vi "Parameter Filter - By Core Number.vi"(2 "Core Number":i32, 7 "Parameters Array (in)":T1[](array[typedef])) -> (8 "Filtered Parameters Array (out)":T1[](array[typedef]))   [LabVIEW 2017] (continued)
 "Scale"="0.5", "Offset"="0", "Signed"=TRUE, "Unit"="Deg C", "Encoding"=enum."BNR", "Default Value"="0"}, {"Core Number"=0, "Channel Number"=7, "Channel Name"="RDC18_ENG_RB1", "Channel Speed"=100, "Label Decimal"=189, "Label Name"="Label_275", "Min Rate (mS)"=800, "Max Rate (mS)"=1200, "SDI"=3, "SSM"=3, "Create SDI"=FALSE, "Create SSM"=FALSE, "Create Parity"=FALSE, "Parameter Name"="rdc18_eng_rb1_lbl275_b18_28", "Start Bit"=18, "Number of Bits"=11, "Scale"="0.5", "Offset"="0", "Signed"=TRUE, "Unit"="Deg C", "Encoding"=enum."BNR", "Default Value"="0"}, {"Core Number"=0, "Channel Number"=7, "Channel Name"="RDC18_ENG_RB1", "Channel Speed"=100, "Label Decimal"=184, "Label Name"="Label_270", "Min Rate (mS)"=80, "Max Rate (mS)"=120, "SDI"=3, "SSM"=0, "Create SDI"=FALSE, "Create SSM"=FALSE, "Create Parity"=FALSE, "Parameter Name"="rdc18_eng_rb1_lbl270_b10_28", "Start Bit"=10, "Number of Bits"=19, "Scale"="1", "Offset"="0", "Signed"=FALSE, "Unit"="N/A", "Encoding"=enum."Discrete", "Default Value"="0"}, {"Core Number"=0, "Channel Number"=7, "Channel Name"="RDC18_ENG_RB1", "Channel Speed"=100, "Label Decimal"=185, "Label Name"="Label_271", "Min Rate (mS)"=80, "Max Rate (mS)"=120, "SDI"=3, "SSM"=0, "Create SDI"=FALSE, "Create SSM"=FALSE, "Create Parity"=FALSE, "Parameter Name"="rdc18_eng_rb1_lbl271_b10_28", "Start Bit"=10, "Number of Bits"=19, "Scale"="1", "Offset"="0", "Signed"=FALSE, "Unit"="N/A", "Encoding"=enum."Discrete", "Default Value"="0"}, {"Core Number"=0, "Channel Number"=7, "Channel Name"="RDC18_ENG_RB1", "Channel Speed"=100, "Label Decimal"=186, "Label Name"="Label_272", "Min Rate (mS)"=80, "Max Rate (mS)"=120, "SDI"=3, "SSM"=0, "Create SDI"=FALSE, "Create SSM"=FALSE, "Create Parity"=FALSE, "Parameter Name"="rdc18_eng_rb1_lbl272_b10_28", "Start Bit"=10, "Number of Bits"=19, "Scale"="1", "Offset"="0", "Signed"=FALSE, "Unit"="N/A", "Encoding"=enum."Discrete", "Default Value"="0"}, {"Core Number"=0, "Channel Number"=7, "Channel Name"="RDC18_ENG_RB1", "Channel Speed"=100, "Label Decimal"=187, "Label Name"="Label_273", "Min Rate (mS)"=80, "Max Rate (mS)"=120, "SDI"=3, "SSM"=0, "Create SDI"=FALSE, "Create SSM"=FALSE, "Create Parity"=FALSE, "Parameter Name"="rdc18_eng_rb1_lbl273_b10_28", "Start Bit"=10, "Number of Bits"=19, "Scale"="1", "Offset"="0", "Signed"=FALSE, "Unit"="N/A", "Encoding"=enum."Discrete", "Default Value"="0"}, {"Core Number"=0, "Channel Number"=7, "Channel Name"="RDC18_ENG_RB1", "Channel Speed"=100, "Label Decimal"=151, "Label Name"="Label_227", "Min Rate (mS)"=80, "Max Rate (mS)"=120, "SDI"=3, "SSM"=0, "Create SDI"=FALSE, "Create SSM"=FALSE, "Create Parity"=FALSE, "Parameter Name"="rdc18_eng_rb1_lbl227_b10_28", "Start Bit"=10, "Number of Bits"=19, "Scale"="1", "Offset"="0", "Signed"=FALSE, "Unit"="N/A", "Encoding"=enum."Discrete", "Default Value"="0"}, {"Core Number"=0, "Channel Number"=7, "Channel Name"="RDC18_ENG_RB1", "Channel Speed"=100, "Label Decimal"=105, "Label Name"="Label_151", "Min Rate (mS)"=800, "Max Rate (mS)"=1200, "SDI"=3, "SSM"=0, "Create SDI"=FALSE, "Create SSM"=FALSE, "Create Parity"=FALSE, "Parameter Name"="rdc18_eng_rb1_lbl151_b10_27", "Start Bit"=10, "Number of Bits"=18, "Scale"="1", "Offset"="0", "Signed"=FALSE, "Unit"="N/A", "Encoding"=enum."Discrete", "Default Value"="0"}, {"Core Number"=0, "Channel Number"=8, "Channel Name"="RDC18_ENG_RB2", "Channel Speed"=100, "Label Decimal"=213, "Label Name"="Label_325", "Min Rate (mS)"=40, "Max Rate (mS)"=60, "SDI"=3, "SSM"=3, "Create SDI"=FALSE, "Create SSM"=FALSE, "Create Parity"=FALSE, "Parameter Name"="rdc18_eng_rb2_lbl325_b10_28", "Start Bit"=10, "Number of Bits"=19, "Scale"="0.0006866", "Offset"="0", "Signed"=TRUE, "Unit"="Degrees", "Encoding"=enum."BNR", "Default Value"="0"}, {"Core Number"=0, "Channel Number"=8, "Channel Name"="RDC18_ENG_RB2", "Channel Speed"=100, "Label Decimal"=91, "Label Name"="Label_133", "Min Rate (mS)"=40, "Max Rate (mS)"=60, "SDI"=3, "SSM"=3, "Create SDI"=FALSE, "Create SSM"=FALSE, "Create Parity"=FALSE, "Parameter Name"="rdc18_eng_rb2_lbl133_b10_28", "Start Bit"=10, "Number of Bits"=19, "Scale"="0.0006866", "Offset"="0", "Signed"=TRUE, "Unit"="Degrees", "Encoding"=enum."BNR", "Default Value"="0"}, {"Core Number"=0, "Channel Number"=8, "Channel Name"="RDC18_ENG_RB2", "Channel Speed"=100, "Label Decimal"=104, "Label Name"="Label_150", "Min Rate (mS)"=800, "Max Rate (mS)"=1200, "SDI"=3, "SSM"=3, "Create SDI"=FALSE, "Create SSM"=FALSE, "Create Parity"=FALSE, "Parameter Name"="rdc18_eng_rb2_lbl150_b11_27", "Start Bit"=11, "Number of Bits"=17, "Scale"="1", "Offset"="0", "Signed"=FALSE, "Unit"="hh.mm.ss", "Encoding"=enum."BNR", "Default Value"="0"}, {"Core Number"=0, "Channel Number"=8, "Channel Name"="RDC18_ENG_RB2", "Channel Speed"=100, "Label Decimal"=39, "Label Name"="Label_47", "Min Rate (mS)"=800, "Max Rate (mS)"=1200, "SDI"=3, "SSM"=3, "Create SDI"=FALSE, "Create SSM"=FALSE, "Create Parity"=FALSE, "Parameter Name"="rdc18_eng_rb2_lbl47_b10_27", "Start Bit"=10, "Number of Bits"=18, "Scale"="1", "Offset"="0", "Signed"=FALSE, "Unit"="N/A", "Encoding"=enum."BNR", "Default Value"="0"}, {"Core Number"=0, "Channel Number"=8, "Channel Name"="RDC18_ENG_RB2", "Channel Speed"=100, "Label Decimal"=188, "Label Name"="Label_274", "Min Rate (mS)"=800, "Max Rate (mS)"=1200, "SDI"=3, "SSM"=3, "Create SDI"=FALSE, "Create SSM"=FALSE, "Create Parity"=FALSE, "Parameter Name"="rdc18_eng_rb2_lbl274_b18_28", "Start Bit"=18, "Number of Bits"=11, "Scale"="0.5", "Offset"="0", "Signed"=TRUE, "Unit"="Deg C", "Encoding"=enum."BNR", "Default Value"="0"}, {"Core Number"=0, "Channel Number"=8, "Channel Name"="RDC18_ENG_RB2", "Channel Speed"=100, "Label Decimal"=189, "Label Name"="Label_275", "Min Rate (mS)"=800, "Max Rate (mS)"=1200, "SDI"=3, "SSM"=3, "Create SDI"=FALSE, "Create SSM"=FALSE, "Create Parity"=FALSE, "Parameter Name"="rdc18_eng_rb2_lbl275_b18_28", "Start Bit"=18, "Number of Bits"=11, "Scale"="0.5", "Offset"="0", "Signed"=TRUE, "Unit"="Deg C", "Encoding"=enum."BNR", "Default Value"="0"}, {"Core Number"=0, "Channel Number"=8, "Channel Name"="RDC18_ENG_RB2", "Channel Speed"=100, "Label Decimal"=184, "Label Name"="Label_270", "Min Rate (mS)"=80, "Max Rate (mS)"=120, "SDI"=3, "SSM"=0, "Create SDI"=FALSE, "Create SSM"=FALSE, "Create Parity"=FALSE, "Parameter Name"="rdc18_eng_rb2_lbl270_b10_28", "Start Bit"=10, "Number of Bits"=19, "Scale"="1", "Offset"="0", "Signed"=FALSE, "Unit"="N/A", "Encoding"=enum."Discrete", "Default Value"="0"}, {"Core Number"=0, "Channel Number"=8, "Channel Name"="RDC18_ENG_RB2", "Channel Speed"=100, "Label Decimal"=185, "Label Name"="Label_271", "Min Rate (mS)"=80, "Max Rate (mS)"=120, "SDI"=3, "SSM"=0, "Create SDI"=FALSE, "Create SSM"=FALSE, "Create Parity"=FALSE, "Parameter Name"="rdc18_eng_rb2_lbl271_b10_28", "Start Bit"=10, "Number of Bits"=19, "Scale"="1", "Offset"="0", "Signed"=FALSE, "Unit"="N/A", "Encoding"=enum."Discrete", "Default Value"="0"}, {"Core Number"=0, "Channel Number"=8, "Channel Name"="RDC18_ENG_RB2", "Channel Speed"=100, "Label Decimal"=186, "Label Name"="Label_272", "Min Rate (mS)"=80, "Max Rate (mS)"=120, "SDI"=3, "SSM"=0, "Create SDI"=FALSE, "Create SSM"=FALSE, "Create Parity"=FALSE, "Parameter Name"="rdc18_eng_rb2_lbl272_b10_28", "Start Bit"=10, "Number of Bits"=19, "Scale"="1", "Offset"="0", "Signed"=FALSE, "Unit"="N/A", "Encoding"=enum."Discrete", "Default Value"="0"}, {"Core Number"=0, "Channel Number"=8, "Channel Name"="RDC18_ENG_RB2", "Channel Speed"=100, "Label Decimal"=187, "Label Name"="Label_273", "Min Rate (mS)"=80, "Max Rate (mS)"=120, "SDI"=3, "SSM"=0, "Create SDI"=FALSE, "Create SSM"=FALSE, "Create Parity"=FALSE, "Parameter Name"="rdc18_eng_rb2_lbl273_b10_28", "Start Bit"=10, "Number of Bits"=19, "Scale"="1", "Offset"="0", "Signed"=FALSE, "Unit"="N/A", "Encoding"=enum."Discrete", "Default Value"="0"}, {"Core Number"=0, "Channel Number"=8, "Channel Name"="RDC18_ENG_RB2", "Channel Speed"=100, "Label Decimal"=151, "Label Name"="Label_227", "Min Rate (mS)"=80, "Max Rate (mS)"=120, "SDI"=3, "SSM"=0, "Create SDI"=FALSE, "Create SSM"=FALSE, "Create Parity"=FALSE, "Parameter Name"="rdc18_eng_rb2_lbl227_b10_28", "Start Bit"=10, "Number of Bits"=19, "Scale"="1", "Offset"="0", "Signed"=FALSE, "Unit"="N/A", "Encoding"=enum."Discrete", "Default Value"="0"}, {"Core Number"=0, "Channel Number"=8, "Channel Name"="RDC18_ENG_RB2", "Channel Speed"=100, "Label Decimal"=105, "Label Name"="Label_151", "Min Rate (mS)"=800, "Max Rate (mS)"=1200, "SDI"=3, "SSM"=0, "Create SDI"=FALSE, "Create SSM"=FALSE, "Create Parity"=FALSE, "Parameter Name"="rdc18_eng_rb2_lbl151_b10_27", "Start Bit"=10, "Number of Bits"=18, "Scale"="1", "Offset"="0", "Signed"=FALSE, "Unit"="N/A", "Encoding"=enum."Discrete", "Default Value"="0"}, {"Core Number"=0, "Channel Number"=27, "Channel Name"="LGCS_MON2_TX", "Channel Speed"=100, "Label Decimal"=17, "Label Name"="Label_21", "Min Rate (mS)"=10, "Max Rate (mS)"=30, "SDI"=0, "SSM"=0, "Create SDI"=FALSE, "Create SSM"=FALSE, "Create Parity"=FALSE, "Parameter Name"="m2_dnlk_status_msg", "Start Bit"=8, "Number of Bits"=23, "Scale"="1", "Offset"="0", "Signed"=FALSE, "Unit"="", "Encoding"=enum."BNR", "Default Value"="0"}, {"Core Number"=0, "Channel Number"=27, "Channel Name"="LGCS_MON2_TX", "Channel Speed"=100, "Label Decimal"=18, "Label Name"="Label_22", "Min Rate (mS)"=10, "Max Rate (mS)"=30, "SDI"=0, "SSM"=0, "Create SDI"=FALSE, "Create SSM"=FALSE, "Create Parity"=FALSE, "Parameter Name"="m2_consilidated_wow_status", "Start Bit"=8, "Number of Bits"=23, "Scale"="1", "Offset"="0", "Signed"=FALSE, "Unit"="", "Encoding"=enum."BNR", "Default Value"="0"}, {"Core Number"=0, "Channel Number"=27, "Channel Name"="LGCS_MON2_TX", "Channel Speed"=100, "Label Decimal"=19, "Label Name"="Label_23", "Min Rate (mS)"=80, "Max Rate (mS)"=120, "SDI"=3, "SSM"=0, "Create SDI"=FALSE, "Create SSM"=FALSE, "Create Parity"=FALSE, "Parameter Name"="baulk_solenoid_ctl_ch1", "Start Bit"=26, "Number of Bits"=1, "Scale"="0", "Offset"="0", "Signed"=FALSE, "Unit"="", "Encoding"=enum."Discrete", "Default Value"="0"}, {"Core Number"=0, "Channel Number"=27, "Channel Name"="LGCS_MON2_TX", "Channel Speed"=100, "Label Decimal"=19, "Label Name"="Label_23", "Min Rate (mS)"=80, "Max Rate (mS)"=120, "SDI"=3, "SSM"=0, "Create SDI"=FALSE, "Create SSM"=FALSE, "Create Parity"=FALSE, "Parameter Name"="baulk_solenoid_ctl_ch2", "Start Bit"=27, "Number of Bits"=1, "Scale"="0", "Offset"="0", "Signed"=FALSE, "Unit"="", "Encoding"=enum."Discrete", "Default Value"="0"}, {"Core Number"=0, "Channel Number"=27, "Channel Name"="LGCS_MON2_TX", "Channel Speed"=100, "Label Decimal"=19, "Label Name"="Label_23", "Min Rate (mS)"=80, "Max Rate (mS)"=120, "SDI"=3, "SSM"=0, "Create SDI"=FALSE, "Create SSM"=FALSE, "Create Parity"=FALSE, "Parameter Name"="mlg_doors_close_highside_solenoid_driver_ctl_ch1", "Start Bit"=17, "Number of Bits"=1, "Scale"="0", "Offset"="0", "Signed"=FALSE, "Unit"="", "Encoding"=enum."Discrete", "Default Value"="0"}, {"Core Number"=0, "Channel Number"=27, "Channel Name"="LGCS_MON2_TX", "Channel Speed"=100, "Label Decimal"=19, "Label Name"="Label_23", "Min Rate (mS)"=80, "Max Rate (mS)"=120, "SDI"=3, "SSM"=0, "Create SDI"=FALSE, "Create SSM"=FALSE, "Create Parity"=FALSE, "Parameter Name"="mlg_doors_close_highside_solenoid_driver_ctl_ch2", "Start Bit"=25, "Number of Bits"=1, "Scale"="0", "Offset"="0", "Signed"=FALSE, "Unit"="", "Encoding"=enum."Discrete", "Default Value"="0"}, {"Core Number"=0, "Channel Number"=27, "Channel Name"="LGCS_MON2_TX", "Channel Speed"=100, "Label Decimal"=19, "Label Name"="Label_23", "Min Rate (mS)"=80, "Max Rate (mS)"=120, "SDI"=3, "SSM"=0, "Create SDI"=FALSE, "Create SSM"=FALSE, "Create Parity"=FALSE, "Parameter Name"="mlg_doors_close_lowside_solenoid_driver_ctl_ch1", "Start Bit"=16, "Number of Bits"=1, "Scale"="0", "Offset"="0", "Signed"=FALSE, "Unit"="", "Encoding"=enum."Discrete", "Default Value"="0"}, {"Core Number"=0, "Channel Number"=27, "Channel Name"="LGCS_MON2_TX", "Channel Speed"=100, "Label Decimal"=19, "Label Name"="Label_23", "Min Rate (mS)"=80, "Max Rate (mS)"=120, "SDI"=3, "SSM"=0, "Create SDI"=FALSE, "Create SSM"=FALSE, "Create Parity"=FALSE, "Parameter Name"="mlg_doors_close_lowside_solenoid_driver_ctl_ch2", "Start Bit"=24, "Number of Bits"=1, "Scale"="0", "Offset"="0", "Signed"=FALSE, "Unit"="", "Encoding"=enum."Discrete", "Default Value"="0"}, {"Core Number"=0, "Channel Number"=27, "Channel Name"="LGCS_MON2_TX", "Channel Speed"=100, "Label Decimal"=19, "Label Name"="Label_23", "Min Rate (mS)"=80, "Max Rate (mS)"=120, "SDI"=3, "SSM"=0, "Create SDI"=FALSE, "Create SSM"=FALSE, "Create Parity"=FALSE, "Parameter Name"="mlg_doors_open_highside_solenoid_driver_ctl_ch1", "Start Bit"=15, "Number of Bits"=1, "Scale"="0", "Offset"="0", "Signed"=FALSE, "Unit"="", "Encoding"=enum."Discrete", "Default Value"="0"}, {"Core Number"=0, "Channel Number"=27, "Channel Name"="LGCS_MON2_TX", "Channel Speed"=100, "Label Decimal"=19, "Label Name"="Label_23", "Min Rate (mS)"=80, "Max Rate (mS)"=120, "SDI"=3, "SSM"=0, "Create SDI"=FALSE, "Create SSM"=FALSE, "Create Parity"=FALSE, "Parameter Name"="mlg_doors_open_highside_solenoid_driver_ctl_ch2", "Start Bit"=23, "Number of Bits"=1, "Scale"="0", "Offset"="0", "Signed"=FALSE, "Unit"="", "Encoding"=enum."Discrete", "Default Value"="0"}, {"Core Number"=0, "Channel Number"=27, "Channel Name"="LGCS_MON2_TX", "Channel Speed"=100, "Label Decimal"=19, "Label Name"="Label_23", "Min Rate (mS)"=80, "Max Rate (mS)"=120, "SDI"=3, "SSM"=0, "Create SDI"=FALSE, "Create SSM"=FALSE, "Create Parity"=FALSE, "Parameter Name"="mlg_doors_open_lowside_solenoid_driver_ctl_ch1", "Start Bit"=14, "Number of Bits"=1, "Scale"="0", "Offset"="0", "Signed"=FALSE, "Unit"="", "Encoding"=enum."Discrete", "Default Value"="0"}, {"Core Number"=0, "Channel Number"=27, "Channel Name"="LGCS_MON2_TX", "Channel Speed"=100, "Label Decimal"=19, "Label Name"="Label_23", "Min Rate (mS)"=80, "Max Rate (mS)"=120, "SDI"=3, "SSM"=0, "Create SDI"=FALSE, "Create SSM"=FALSE, "Create Parity"=FALSE, "Parameter Name"="mlg_doors_open_lowside_solenoid_driver_ctl_ch2", "Start Bit"=22, "Number of Bits"=1, "Scale"="0", "Offset"="0", "Signed"=FALSE, "Unit"="", "Encoding"=enum."Discrete", "Default Value"="0"}, {"Core Number"=0, "Channel Number"=27, "Channel Name"="LGCS_MON2_TX", "Channel Speed"=100, "Label Decimal"=19, "Label Name"="Label_23", "Min Rate (mS)"=80, "Max Rate (mS)"=120, "SDI"=3, "SSM"=0, "Create SDI"=FALSE, "Create SSM"=FALSE, "Create Parity"=FALSE, "Parameter Name"="mlg_extend_highsidesolenoiddriver_ctl_ch1", "Start Bit"=13, "Number of Bits"=1, "Scale"="0", "Offset"="0", "Signed"=FALSE, "Unit"="", "Encoding"=enum."Discrete", "Default Value"="0"}, {"Core Number"=0, "Channel Number"=27, "Channel Name"="LGCS_MON2_TX", "Channel Speed"=100, "Label Decimal"=19, "Label Name"="Label_23", "Min Rate (mS)"=80, "Max Rate (mS)"=120, "SDI"=3, "SSM"=0, "Create SDI"=FALSE, "Create SSM"=FALSE, "Create Parity"=FALSE, "Parameter Name"="mlg_extend_highsidesolenoiddriver_ctl_ch2", "Start Bit"=21, "Number of Bits"=1, "Scale"="0", "Offset"="0", "Signed"=FALSE, "Unit"="", "Encoding"=enum."Discrete", "Default Value"="0"}, {"Core Number"=0, "Channel Number"=27, "Channel Name"="LGCS_MON2_TX", "Channel Speed"=100, "Label Decimal"=19, "Label Name"="Label_23", "Min Rate (mS)"=80, "Max Rate (mS)"=120, "SDI"=3, "SSM"=0, "Create SDI"=FALSE, "Create SSM"=FALSE, "Create Parity"=FALSE, "Parameter Name"="mlg_extend_lowsidesolenoiddriver_ctl_ch1", "Start Bit"=12, "Number of Bits"=1, "Scale"="0", "Offset"="0", "Signed"=FALSE, "Unit"="", "Encoding"=enum."Discrete", "Default Value"="0"}, {"Core Number"=0, "Channel Number"=27, "Channel Name"="LGCS_MON2_TX", "Channel Speed"=100, "Label Decimal"=19, "Label Name"="Label_23", "Min Rate (mS)"=80, "Max Rate (mS)"=120, "SDI"=3, "SSM"=0, "Create SDI"=FALSE, "Create SSM"=FALSE, "Create Parity"=FALSE, "Parameter Name"="mlg_extend_lowsidesolenoiddriver_ctl_ch2", "Start Bit"=20, "Number of Bits"=1, "Scale"="0", "Offset"="0", "Signed"=FALSE, "Unit"="", "Encoding"=enum."Discrete", "Default Value"="0"}, {"Core Number"=0, "Channel Number"=27, "Channel Name"="LGCS_MON2_TX", "Channel Speed"=100, "Label Decimal"=19, "Label Name"="Label_23", "Min Rate (mS)"=80, "Max Rate (mS)"=120, "SDI"=3, "SSM"=0, "Create SDI"=FALSE, "Create SSM"=FALSE, "Create Parity"=FALSE, "Parameter Name"="mlg_retract_highsidesolenoiddriver_ctl_ch1", "Start Bit"=11, "Number of Bits"=1, "Scale"="0", "Offset"="0", "Signed"=FALSE, "Unit"="", "Encoding"=enum."Discrete", "Default Value"="0"}, {"Core Number"=0, "Channel Number"=27, "Channel Name"="LGCS_MON2_TX", "Channel Speed"=100, "Label Decimal"=19, "Label Name"="Label_23", "Min Rate (mS)"=80, "Max Rate (mS)"=120, "SDI"=3, "SSM"=0, "Create SDI"=FALSE, "Create SSM"=FALSE, "Create Parity"=FALSE, "Parameter Name"="mlg_retract_highsidesolenoiddriver_ctl_ch2", "Start Bit"=19, "Number of Bits"=1, "Scale"="0", "Offset"="0", "Signed"=FALSE, "Unit"="", "Encoding"=enum."Discrete", "Default Value"="0"}, {"Core Number"=0, "Channel Number"=27, "Channel Name"="LGCS_MON2_TX", "Channel Speed"=100, "Label Decimal"=19, "Label Name"="Label_23", "Min Rate (mS)"=80, "Max Rate (mS)"=120, "SDI"=3, "SSM"=0, "Create SDI"=FALSE, "Create SSM"=FALSE, "Create Parity"=FALSE, "Parameter Name"="mlg_retract_lowsidesolenoiddriver_ctl_ch1", "Start Bit"=10, "Number of Bits"=1, "Scale"="0", "Offset"="0", "Signed"=FALSE, "Unit"="", "Encoding"=enum."Discrete", "Default Value"="0"}, {"Core Number"=0, "Channel Number"=27, "Channel Name"="LGCS_MON2_TX", "Channel Speed"=100, "Label Decimal"=19, "Label Name"="Label_23", "Min Rate (mS)"=80, "Max Rate (mS)"=120, "SDI"=3, "SSM"=0, "Create SDI"=FALSE, "Create SSM"=FALSE, "Create Parity"=FALSE, "Parameter Name"="mlg_retract_lowsidesolenoiddriver_ctl_ch2", "Start Bit"=18, "Number of Bits"=1, "Scale"="0", "Offset"="0", "Signed"=FALSE, "Unit"="", "Encoding"=enum."Discrete", "Default Value"="0"}, {"Core Number"=0, "Channel Number"=27, "Channel Name"="LGCS_MON2_TX", "Channel Speed"=100, "Label Decimal"=20, "Label Name"="Label_24", "Min Rate (mS)"=80, "Max Rate (mS)"=120, "SDI"=0, "SSM"=0, "Create SDI"=FALSE, "Create SSM"=FALSE, "Create Parity"=FALSE, "Parameter Name"="m1_m2_cas_msg", "Start Bit"=8, "Number of Bits"=23, "Scale"="1", "Offset"="0", "Signed"=FALSE, "Unit"="", "Encoding"=enum."BNR", "Default Value"="0"}, {"Core Number"=0, "Channel Number"=27, "Channel Name"="LGCS_MON2_TX", "Channel Speed"=100, "Label Decimal"=21, "Label Name"="Label_25", "Min Rate (mS)"=80, "Max Rate (mS)"=120, "SDI"=3, "SSM"=0, "Create SDI"=FALSE, "Create SSM"=FALSE, "Create Parity"=FALSE, "Parameter Name"="baulk_solenoid_ctl_ch1", "Start Bit"=26, "Number of Bits"=1, "Scale"="0", "Offset"="0", "Signed"=FALSE, "Unit"="", "Encoding"=enum."Discrete", "Default Value"="0"}, {"Core Number"=0, "Channel Number"=27, "Channel Name"="LGCS_MON2_TX", "Channel Speed"=100, "Label Decimal"=21, "Label Name"="Label_25", "Min Rate (mS)"=80, "Max Rate (mS)"=120, "SDI"=3, "SSM"=0, "Create SDI"=FALSE, "Create SSM"=FALSE, "Create Parity"=FALSE, "Parameter Name"="baulk_solenoid_ctl_ch2", "Start Bit"=27, "Number of Bits"=1, "Scale"="0", "Offset"="0", "Signed"=FALSE, "Unit"="", "Encoding"=enum."Discrete", "Default Value"="0"}, {"Core Number"=0, "Channel Number"=27, "Channel Name"="LGCS_MON2_TX", "Channel Speed"=100, "Label Decimal"=21, "Label Name"="Label_25", "Min Rate (mS)"=80, "Max Rate (mS)"=120, "SDI"=3, "SSM"=0, "Create SDI"=FALSE, "Create SSM"=FALSE, "Create Parity"=FALSE, "Parameter Name"="nlg_doors_close_highside_solenoid_driver_ctl_ch1", "Start Bit"=17, "Number of Bits"=1, "Scale"="0", "Offset"="0", "Signed"=FALSE, "Unit"="", "Encoding"=enum."Discrete", "Default Value"="0"}, {"Core Number"=0, "Channel Number"=27, "Channel Name"="LGCS_MON2_TX", "Channel Speed"=100, "Label Decimal"=21, "Label Name"="Label_25", "Min Rate (mS)"=80, "Max Rate (mS)"=120, "SDI"=3, "SSM"=0, "Create SDI"=FALSE, "Create SSM"=FALSE, "Create Parity"=FALSE, "Parameter Name"="nlg_doors_close_highside_solenoid_driver_ctl_ch2", "Start Bit"=25, "Number of Bits"=1, "Scale"="0", "Offset"="0", "Signed"=FALSE, "Unit"="", "Encoding"=enum."Discrete", "Default Value"="0"}, {"Core Number"=0, "Channel Number"=27, "Channel Name"="LGCS_MON2_TX", "Channel Speed"=100, "Label Decimal"=21, "Label Name"="Label_25", "Min Rate (mS)"=80, "Max Rate (mS)"=120, "SDI"=3, "SSM"=0, "Create SDI"=FALSE, "Create SSM"=FALSE, "Create Parity"=FALSE, "Parameter Name"="nlg_doors_close_lowside_solenoid_driver_ctl_ch1", "Start Bit"=16, "Number of Bits"=1, "Scale"="0", "Offset"="0", "Signed"=FALSE, "Unit"="", "Encoding"=enum."Discrete", "Default Value"="0"}, {"Core Number"=0, "Channel Number"=27, "Channel Name"="LGCS_MON2_TX", "Channel Speed"=100, "Label Decimal"=21, "Label Name"="Label_25", "Min Rate (mS)"=80, "Max Rate (mS)"=120, "SDI"=3, "SSM"=0, "Create SDI"=FALSE, "Create SSM"=FALSE, "Create Parity"=FALSE, "Parameter Name"="nlg_doors_close_lowside_solenoid_driver_ctl_ch2", "Start Bit"=24, "Number of Bits"=1, "Scale"="0", "Offset"="0", "Signed"=FALSE, "Unit"="", "Encoding"=enum."Discrete", "Default Value"="0"}, {"Core Number"=0, "Channel Number"=27, "Channel Name"="LGCS_MON2_TX", "Channel Speed"=100, "Label Decimal"=21, "Label Name"="Label_25", "Min Rate (mS)"=80, "Max Rate (mS)"=120, "SDI"=3, "SSM"=0, "Create SDI"=FALSE, "Create SSM"=FALSE, "Create Parity"=FALSE, "Parameter Name"="nlg_doors_open_highside_solenoid_driver_ctl_ch1", "Start Bit"=15, "Number of Bits"=1, "Scale"="0", "Offset"="0", "Signed"=FALSE, "Unit"="", "Encoding"=enum."Discrete", "Default Value"="0"}, {"Core Number"=0, "Channel Number"=27, "Channel Name"="LGCS_MON2_TX", "Channel Speed"=100, "Label Decimal"=21, "Label Name"="Label_25", "Min Rate (mS)"=80, "Max Rate (mS)"=120, "SDI"=3, "SSM"=0, "Create SDI"=FALSE, "Create SSM"=FALSE, "Create Parity"=FALSE, "Parameter Name"="nlg_doors_open_highside_solenoid_driver_ctl_ch2", "Start Bit"=23, "Number of Bits"=1, "Scale"="0", "Offset"="0", "Signed"=FALSE, "Unit"="", "Encoding"=enum."Discrete", "Default Value"="0"}, {"Core Number"=0, "Channel Number"=27, "Channel Name"="LGCS_MON2_TX", "Channel Speed"=100, "Label Decimal"=21, "Label Name"="Label_25", "Min Rate (mS)"=80, "Max Rate (mS)"=120, "SDI"=3, "SSM"=0, "Create SDI"=FALSE, "Create SSM"=FALSE, "Create Parity"=FALSE, "Parameter Name"="nlg_doors_open_lowside_solenoid_driver_ctl_ch1", "Start Bit"=14, "Number of Bits"=1, "Scale"="0", "Offset"="0", "Signed"=FALSE, "Unit"="", "Encoding"=enum."Discrete", "Default Value"="0"}, {"Core Number"=0, "Channel Number"=27, "Channel Name"="LGCS_MON2_TX", "Channel Speed"=100, "Label Decimal"=21, "Label Name"="Label_25", "Min Rate (mS)"=80, "Max Rate (mS)"=120, "SDI"=3, "SSM"=0, "Create SDI"=FALSE, "Create SSM"=FALSE, "Create Parity"=FALSE, "Parameter Name"="nlg_doors_open_lowside_solenoid_driver_ctl_ch2", "Start Bit"=22, "Number of Bits"=1, "Scale"="0", "Offset"="0", "Signed"=FALSE, "Unit"="", "Encoding"=enum."Discrete", "Default Value"="0"}, {"Core Number"=0, "Channel Number"=27, "Channel Name"="LGCS_MON2_TX", "Channel Speed"=100, "Label Decimal"=21, "Label Name"="Label_25", "Min Rate (mS)"=80, "Max Rate (mS)"=120, "SDI"=3, "SSM"=0, "Create SDI"=FALSE, "Create SSM"=FALSE, "Create Parity"=FALSE, "Parameter Name"="nlg_extend_highsidesolenoiddriver_ctl_ch1", "Start Bit"=13, "Number of Bits"=1, "Scale"="0", "Offset"="0", "Signed"=FALSE, "Unit"="", "Encoding"=enum."Discrete", "Default Value"="0"}, {"Core Number"=0, "Channel Number"=27, "Channel Name"="LGCS_MON2_TX", "Channel Speed"=100, "Label Decimal"=21, "Label Name"="Label_25", "Min Rate (mS)"=80, "Max Rate (mS)"=120, "SDI"=3, "SSM"=0, "Create SDI"=FALSE, "Create SSM"=FALSE, "Create Parity"=FALSE, "Parameter Name"="nlg_extend_highsidesolenoiddriver_ctl_ch2", "Start Bit"=21, "Number of Bits"=1, "Scale"="0", "Offset"="0", "Signed"=FALSE, "Unit"="", "Encoding"=enum."Discrete", "Default Value"="0"}, {"Core Number"=0, "Channel Number"=27, "Channel Name"="LGCS_MON2_TX", "Channel Speed"=100, "Label Decimal"=21, "Label Name"="Label_25", "Min Rate (mS)"=80, "Max Rate (mS)"=120, "SDI"=3, "SSM"=0, "Create SDI"=FALSE, "Create SSM"=FALSE, "Create Parity"=FALSE, "Parameter Name"="nlg_extend_lowsidesolenoiddriver_ctl_ch1", "Start Bit"=12, "Number of Bits"=1, "Scale"="0", "Offset"="0", "Signed"=FALSE, "Unit"="", "Encoding"=enum."Discrete", "Default Value"="0"}, {"Core Number"=0, "Channel Number"=27, "Channel Name"="LGCS_MON2_TX", "Channel Speed"=100, "Label Decimal"=21, "Label Name"="Label_25", "Min Rate (mS)"=80, "Max Rate (mS)"=120, "SDI"=3, "SSM"=0, "Create SDI"=FALSE, "Create SSM"=FALSE, "Create Parity"=FALSE, "Parameter Name"="nlg_extend_lowsidesolenoiddriver_ctl_ch2", "Start Bit"=20, "Number of Bits"=1, "Scale"="0", "Offset"="0", "Signed"=FALSE, "Unit"="", "Encoding"=enum."Discrete", "Default Value"="0"}, {"Core Number"=0, "Channel Number"=27, "Channel Name"="LGCS_MON2_TX", "Channel Speed"=100, "Label Decimal"=21, "Label Name"="Label_25", "Min Rate (mS)"=80, "Max Rate (mS)"=120, "SDI"=3, "SSM"=0, "Create SDI"=FALSE, "Create SSM"=FALSE, "Create Parity"=FALSE, "Parameter Name"="nlg_retract_highsidesolenoiddriver_ctl_ch1", "Start Bit"=11, "Number of Bits"=1, "Scale"="0", "Offset"="0", "Signed"=FALSE, "Unit"="", "Encoding"=enum."Discrete", "Default Value"="0"}, {"Core Number"=0, "Channel Number"=27, "Channel Name"="LGCS_MON2_TX", "Channel Speed"=100, "Label Decimal"=21, "Label Name"="Label_25", "Min Rate (mS)"=80, "Max Rate (mS)"=120, "SDI"=3, "SSM"=0, "Create SDI"=FALSE, "Create SSM"=FALSE, "Create Parity"=FALSE, "Parameter Name"="nlg_retract_highsidesolenoiddriver_ctl_ch2", "Start Bit"=19, "Number of Bits"=1, "Scale"="0", "Offset"="0", "Signed"=FALSE, "Unit"="", "Encoding"=enum."Discrete", "Default Value"="0"}, {"Core Number"=0, "Channel Number"=27, "Channel Name"="LGCS_MON2_TX", "Channel Speed"=100, "Label Decimal"=21, "Label Name"="Label_25", "Min Rate (mS)"=80, "Max Rate (mS)"=120, "SDI"=3, "SSM"=0, "Create SDI"=FALSE, "Create SSM"=FALSE, "Create Parity"=FALSE, "Parameter Name"="nlg_retract_lowsidesolenoiddriver_ctl_ch1", "Start Bit"=10, "Number of Bits"=1, "Scale"="0", "Offset"="0", "Signed"=FALSE, "Unit"="", "Encoding"=enum."Discrete", "Default Value"="0"}, {"Core Number"=0, "Channel Number"=27, "Channel Name"="LGCS_MON2_TX", "Channel Speed"=100, "Label Decimal"=21, "Label Name"="Label_25", "Min Rate (mS)"=80, "Max Rate (mS)"=120, "SDI"=3, "SSM"=0, "Create SDI"=FALSE, "Create SSM"=FALSE, "Create Parity"=FALSE, "Parameter Name"="nlg_retract_lowsidesolenoiddriver_ctl_ch2", "Start Bit"=18, "Number of Bits"=1, "Scale"="0", "Offset"="0", "Signed"=FALSE, "Unit"="", "Encoding"=enum."Discrete", "Default Value"="0"}, {"Core Number"=0, "Channel Number"=27, "Channel Name"="LGCS_MON2_TX", "Channel Speed"=100, "Label Decimal"=22, "Label Name"="Label_26", "Min Rate (mS)"=10, "Max Rate (mS)"=30, "SDI"=0, "SSM"=0, "Create SDI"=FALSE, "Create SSM"=FALSE, "Create Parity"=FALSE, "Parameter Name"="wow_status_and_health_msg", "Start Bit"=8, "Number of Bits"=23, "Scale"="1", "Offset"="0", "Signed"=FALSE, "Unit"="", "Encoding"=enum."BNR", "Default Value"="0"}, {"Core Number"=0, "Channel Number"=27, "Channel Name"="LGCS_MON2_TX", "Channel Speed"=100, "Label Decimal"=32, "Label Name"="Label_40", "Min Rate (mS)"=320, "Max Rate (mS)"=480, "SDI"=2, "SSM"=0, "Create SDI"=FALSE, "Create SSM"=FALSE, "Create Parity"=FALSE, "Parameter Name"="mlg1_lh_door_closed_0_0_0_0_1_1", "Start Bit"=12, "Number of Bits"=1, "Scale"="0", "Offset"="0", "Signed"=FALSE, "Unit"="", "Encoding"=enum."Discrete", "Default Value"="0"}, {"Core Number"=0, "Channel Number"=27, "Channel Name"="LGCS_MON2_TX", "Channel Speed"=100, "Label Decimal"=32, "Label Name"="Label_40", "Min Rate (mS)"=320, "Max Rate (mS)"=480, "SDI"=2, "SSM"=0, "Create SDI"=FALSE, "Create SSM"=FALSE, "Create Parity"=FALSE, "Parameter Name"="mlg1_lh_door_closed_0_0_1_1_0_0", "Start Bit"=11, "Number of Bits"=1, "Scale"="0", "Offset"="0", "Signed"=FALSE, "Unit"="", "Encoding"=enum."Discrete", "Default Value"="0"}, {"Core Number"=0, "Channel Number"=27, "Channel Name"="LGCS_MON2_TX", "Channel Speed"=100, "Label Decimal"=32, "Label Name"="Label_40", "Min Rate (mS)"=320, "Max Rate (mS)"=480, "SDI"=2, "SSM"=0, "Create SDI"=FALSE, "Create SSM"=FALSE, "Create Parity"=FALSE, "Parameter Name"="mlg1_lh_door_closed_0_1_0_1_0_1", "Start Bit"=10, "Number of Bits"=1, "Scale"="0", "Offset"="0", "Signed"=FALSE, "Unit"="", "Encoding"=enum."Discrete", "Default Value"="0"}, {"Core Number"=0, "Channel Number"=27, "Channel Name"="LGCS_MON2_TX", "Channel Speed"=100, "Label Decimal"=32, "Label Name"="Label_40", "Min Rate (mS)"=320, "Max Rate (mS)"=480, "SDI"=2, "SSM"=0, "Create SDI"=FALSE, "Create SSM"=FALSE, "Create Parity"=FALSE, "Parameter Name"="mlg1_lh_door_closed_acid_0_0_0_1___g650_g71_g72_g73", "Start Bit"=15, "Number of Bits"=1, "Scale"="0", "Offset"="0", "Signed"=FALSE, "Unit"="", "Encoding"=enum."Discrete", "Default Value"="0"}, {"Core Number"=0, "Channel Number"=27, "Channel Name"="LGCS_MON2_TX", "Channel Speed"=100, "Label Decimal"=32, "Label Name"="Label_40", "Min Rate (mS)"=320, "Max Rate (mS)"=480, "SDI"=2, "SSM"=0, "Create SDI"=FALSE, "Create SSM"=FALSE, "Create Parity"=FALSE, "Parameter Name"="mlg1_lh_door_closed_acid_0_0_1_1___g650_g71_g72_g73", "Start Bit"=14, "Number of Bits"=1, "Scale"="0", "Offset"="0", "Signed"=FALSE, "Unit"="", "Encoding"=enum."Discrete", "Default Value"="0"}, {"Core Number"=0, "Channel Number"=27, "Channel Name"="LGCS_MON2_TX", "Channel Speed"=100, "Label Decimal"=32, "Label Name"="Label_40", "Min Rate (mS)"=320, "Max Rate (mS)"=480, "SDI"=2, "SSM"=0, "Create SDI"=FALSE, "Create SSM"=FALSE, "Create Parity"=FALSE, "Parameter Name"="mlg1_lh_door_closed_acid_0_1_0_0___g650_g71_g72_g73", "Start Bit"=13, "Number of Bits"=1, "Scale"="0", "Offset"="0", "Signed"=FALSE, "Unit"="", "Encoding"=enum."Discrete", "Default Value"="0"}, {"Core Number"=0, "Channel Number"=27, "Channel Name"="LGCS_MON2_TX", "Channel Speed"=100, "Label Decimal"=32, "Label Name"="Label_40", "Min Rate (mS)"=320, "Max Rate (mS)"=480, "SDI"=2, "SSM"=0, "Create SDI"=FALSE, "Create SSM"=FALSE, "Create Parity"=FALSE, "Parameter Name"="mlg1_lh_door_closed_prox_sensor_trend_available", "Start Bit"=23, "Number of Bits"=1, "Scale"="0", "Offset"="0", "Signed"=FALSE, "Unit"="", "Encoding"=enum."Discrete", "Default Value"="0"}, {"Core Number"=0, "Channel Number"=27, "Channel Name"="LGCS_MON2_TX", "Channel Speed"=100, "Label Decimal"=32, "Label Name"="Label_40", "Min Rate (mS)"=320, "Max Rate (mS)"=480, "SDI"=2, "SSM"=0, "Create SDI"=FALSE, "Create SSM"=FALSE, "Create Parity"=FALSE, "Parameter Name"="mlg1_lh_door_closed_prox_sensor_trend_mon_info_lsb", "Start Bit"=16, "Number of Bits"=1, "Scale"="0", "Offset"="0", "Signed"=FALSE, "Unit"="", "Encoding"=enum."Discrete", "Default Value"="0"}, {"Core Number"=0, "Channel Number"=27, "Channel Name"="LGCS_MON2_TX", "Channel Speed"=100, "Label Decimal"=32, "Label Name"="Label_40", "Min Rate (mS)"=320, "Max Rate (mS)"=480, "SDI"=2, "SSM"=0, "Create SDI"=FALSE, "Create SSM"=FALSE, "Create Parity"=FALSE, "Parameter Name"="mlg1_lh_door_closed_prox_sensor_trend_mon_info_lsb1", "Start Bit"=17, "Number of Bits"=1, "Scale"="0", "Offset"="0", "Signed"=FALSE, "Unit"="", "Encoding"=enum."Discrete", "Default Value"="0"}, {"Core Number"=0, "Channel Number"=27, "Channel Name"="LGCS_MON2_TX", "Channel Speed"=100, "Label Decimal"=32, "Label Name"="Label_40", "Min Rate (mS)"=320, "Max Rate (mS)"=480, "SDI"=2, "SSM"=0, "Create SDI"=FALSE, "Create SSM"=FALSE, "Create Parity"=FALSE, "Parameter Name"="mlg1_lh_door_closed_prox_sensor_trend_mon_info_lsb2", "Start Bit"=18, "Number of Bits"=1, "Scale"="0", "Offset"="0", "Signed"=FALSE, "Unit"="", "Encoding"=enum."Discrete", "Default Value"="0"}, {"Core Number"=0, "Channel Number"=27, "Channel Name"="LGCS_MON2_TX", "Channel Speed"=100, "Label Decimal"=32, "Label Name"="Label_40", "Min Rate (mS)"=320, "Max Rate (mS)"=480, "SDI"=2, "SSM"=0, "Create SDI"=FALSE, "Create SSM"=FALSE, "Create Parity"=FALSE, "Parameter Name"="mlg1_lh_door_closed_prox_sensor_trend_mon_info_lsb3", "Start Bit"=19, "Number of Bits"=1, "Scale"="0", "Offset"="0", "Signed"=FALSE, "Unit"="", "Encoding"=enum."Discrete", "Default Value"="0"}, {"Core Number"=0, "Channel Number"=27, "Channel Name"="LGCS_MON2_TX", "Channel Speed"=100, "Label Decimal"=32, "Label Name"="Label_40", "Min Rate (mS)"=320, "Max Rate (mS)"=480, "SDI"=2, "SSM"=0, "Create SDI"=FALSE, "Create SSM"=FALSE, "Create Parity"=FALSE, "Parameter Name"="mlg1_lh_door_closed_prox_sensor_trend_mon_info_lsb4", "Start Bit"=20, "Number of Bits"=1, "Scale"="0", "Offset"="0", "Signed"=FALSE, "Unit"="", "Encoding"=enum."Discrete", "Default Value"="0"}, {"Core Number"=0, "Channel Number"=27, "Channel Name"="LGCS_MON2_TX", "Channel Speed"=100, "Label Decimal"=32, "Label Name"="Label_40", "Min Rate (mS)"=320, "Max Rate (mS)"=480, "SDI"=2, "SSM"=0, "Create SDI"=FALSE, "Create SSM"=FALSE, "Create Parity"=FALSE, "Parameter Name"="mlg1_lh_door_closed_prox_sensor_trend_mon_info_lsb5", "Start Bit"=21, "Number of Bits"=1, "Scale"="0", "Offset"="0", "Signed"=FALSE, "Unit"="", "Encoding"=enum."Discrete", "Default Value"="0"}, {"Core Number"=0, "Channel Number"=27, "Channel Name"="LGCS_MON2_TX", "Channel Speed"=100, "Label Decimal"=32, "Label Name"="Label_40", "Min Rate (mS)"=320, "Max Rate (mS)"=480, "SDI"=2, "SSM"=0, "Create SDI"=FALSE, "Create SSM"=FALSE, "Create Parity"=FALSE, "Parameter Name"="mlg1_lh_door_closed_prox_sensor_trend_mon_info_msb", "Start Bit"=22, "Number of Bits"=1, "Scale"="0", "Offset"="0", "Signed"=FALSE, "Unit"="", "Encoding"=enum."Discrete", "Default Value"="0"}, {"Core Number"=0, "Channel Number"=27, "Channel Name"="LGCS_MON2_TX", "Channel Speed"=100, "Label Decimal"=32, "Label Name"="Label_40", "Min Rate (mS)"=320, "Max Rate (mS)"=480, "SDI"=1, "SSM"=0, "Create SDI"=FALSE, "Create SSM"=FALSE, "Create Parity"=FALSE, "Parameter Name"="mlg1_lh_door_closed_0_0_0_0_1_11", "Start Bit"=12, "Number of Bits"=1, "Scale"="0", "Offset"="0", "Signed"=FALSE, "Unit"="", "Encoding"=enum."Discrete", "Default Value"="0"}, {"Core Number"=0, "Channel Number"=27, "Channel Name"="LGCS_MON2_TX", "Channel Speed"=100, "Label Decimal"=32, "Label Name"="Label_40", "Min Rate (mS)"=320, "Max Rate (mS)"=480, "SDI"=1, "SSM"=0, "Create SDI"=FALSE, "Create SSM"=FALSE, "Create Parity"=FALSE, "Parameter Name"="mlg1_lh_door_closed_0_0_1_1_0_01", "Start Bit"=11, "Number of Bits"=1, "Scale"="0", "Offset"="0", "Signed"=FALSE, "Unit"="", "Encoding"=enum."Discrete", "Default Value"="0"}, {"Core Number"=0, "Channel Number"=27, "Channel Name"="LGCS_MON2_TX", "Channel Speed"=100, "Label Decimal"=32, "Label Name"="Label_40", "Min Rate (mS)"=320, "Max Rate (mS)"=480, "SDI"=1, "SSM"=0, "Create SDI"=FALSE, "Create SSM"=FALSE, "Create Parity"=FALSE, "Parameter Name"="mlg1_lh_door_closed_0_1_0_1_0_11", "Start Bit"=10, "Number of Bits"=1, "Scale"="0", "Offset"="0", "Signed"=FALSE, "Unit"="", "Encoding"=enum."Discrete", "Default Value"="0"}, {"Core Number"=0, "Channel Number"=27, "Channel Name"="LGCS_MON2_TX", "Channel Speed"=100, "Label Decimal"=32, "Label Name"="Label_40", "Min Rate (mS)"=320, "Max Rate (mS)"=480, "SDI"=1, "SSM"=0, "Create SDI"=FALSE, "Create SSM"=FALSE, "Create Parity"=FALSE, "Parameter Name"="mlg1_lh_door_closed_acid_0_0_0_1___g650_g71_g72_g731", "Start Bit"=15, "Number of Bits"=1, "Scale"="0", "Offset"="0", "Signed"=FALSE, "Unit"="", "Encoding"=enum."Discrete", "Default Value"="0"}, {"Core Number"=0, "Channel Number"=27, "Channel Name"="LGCS_MON2_TX", "Channel Speed"=100, "Label Decimal"=32, "Label Name"="Label_40", "Min Rate (mS)"=320, "Max Rate (mS)"=480, "SDI"=1, "SSM"=0, "Create SDI"=FALSE, "Create SSM"=FALSE, "Create Parity"=FALSE, "Parameter Name"="mlg1_lh_door_closed_acid_0_0_1_1___g650_g71_g72_g731", "Start Bit"=14, "Number of Bits"=1, "Scale"="0", "Offset"="0", "Signed"=FALSE, "Unit"="", "Encoding"=enum."Discrete", "Default Value"="0"}, {"Core Number"=0, "Channel Number"=27, "Channel Name"="LGCS_MON2_TX", "Channel Speed"=100, "Label Decimal"=32, "Label Name"="Label_40", "Min Rate (mS)"=320, "Max Rate (mS)"=480, "SDI"=1, "SSM"=0, "Create SDI"=FALSE, "Create SSM"=FALSE, "Create Parity"=FALSE, "Parameter Name"="mlg1_lh_door_closed_acid_0_1_0_0___g650_g71_g72_g731", "Start Bit"=13, "Number of Bits"=1, "Scale"="0", "Offset"="0", "Signed"=FALSE, "Unit"="", "Encoding"=enum."Discrete", "Default Value"="0"}, {"Core Number"=0, "Channel Number"=27, "Channel Name"="LGCS_MON2_TX", "Channel Speed"=100, "Label Decimal"=32, "Label Name"="Label_40", "Min Rate (mS)"=320, "Max Rate (mS)"=480, "SDI"=1, "SSM"=0, "Create SDI"=FALSE, "Create SSM"=FALSE, "Create Parity"=FALSE, "Parameter Name"="mlg1_lh_door_closed_prox_sensor_trend_available1", "Start Bit"=23, "Number of Bits"=1, "Scale"="0", "Offset"="0", "Signed"=FALSE, "Unit"="", "Encoding"=enum."Discrete", "Default Value"="0"}, {"Core Number"=0, "Channel Number"=27, "Channel Name"="LGCS_MON2_TX", "Channel Speed"=100, "Label Decimal"=32, "Label Name"="Label_40", "Min Rate (mS)"=320, "Max Rate (mS)"=480, "SDI"=1, "SSM"=0, "Create SDI"=FALSE, "Create SSM"=FALSE, "Create Parity"=FALSE, "Parameter Name"="mlg1_lh_door_closed_prox_sensor_trend_mon_info_lsb1", "Start Bit"=16, "Number of Bits"=1, "Scale"="0", "Offset"="0", "Signed"=FALSE, "Unit"="", "Encoding"=enum."Discrete", "Default Value"="0"}, {"Core Number"=0, "Channel Number"=27, "Channel Name"="LGCS_MON2_TX", "Channel Speed"=100, "Label Decimal"=32, "Label Name"="Label_40", "Min Rate (mS)"=320, "Max Rate (mS)"=480, "SDI"=1, "SSM"=0, "Create SDI"=FALSE, "Create SSM"=FALSE, "Create Parity"=FALSE, "Parameter Name"="mlg1_lh_door_closed_prox_sensor_trend_mon_info_lsb11", "Start Bit"=17, "Number of Bits"=1, "Scale"="0", "Offset"="0", "Signed"=FALSE, "Unit"="", "Encoding"=enum."Discrete", "Default Value"="0"}, {"Core Number"=0, "Channel Number"=27, "Channel Name"="LGCS_MON2_TX", "Channel Speed"=100, "Label Decimal"=32, "Label Name"="Label_40", "Min Rate (mS)"=320, "Max Rate (mS)"=480, "SDI"=1, "SSM"=0, "Create SDI"=FALSE, "Create SSM"=FALSE, "Create Parity"=FALSE, "Parameter Name"="mlg1_lh_door_closed_prox_sensor_trend_mon_info_lsb21", "Start Bit"=18, "Number of Bits"=1, "Scale"="0", "Offset"="0", "Signed"=FALSE, "Unit"="", "Encoding"=enum."Discrete", "Default Value"="0"}, {"Core Number"=0, "Channel Number"=27, "Channel Name"="LGCS_MON2_TX", "Channel Speed"=100, "Label Decimal"=32, "Label Name"="Label_40", "Min Rate (mS)"=320, "Max Rate (mS)"=480, "SDI"=1, "SSM"=0, "Create SDI"=FALSE, "Create SSM"=FALSE, "Create Parity"=FALSE, "Parameter Name"="mlg1_lh_door_closed_prox_sensor_trend_mon_info_lsb31", "Start Bit"=19, "Number of Bits"=1, "Scale"="0", "Offset"="0", "Signed"=FALSE, "Unit"="", "Encoding"=enum."Discrete", "Default Value"="0"}, {"Core Number"=0, "Channel Number"=27, "Channel Name"="LGCS_MON2_TX", "Channel Speed"=100, "Label Decimal"=32, "Label Name"="Label_40", "Min Rate (mS)"=320, "Max Rate (mS)"=480, "SDI"=1, "SSM"=0, "Create SDI"=FALSE, "Create SSM"=FALSE, "Create Parity"=FALSE, "Parameter Name"="mlg1_lh_door_closed_prox_sensor_trend_mon_info_lsb41", "Start Bit"=20, "Number of Bits"=1, "Scale"="0", "Offset"="0", "Signed"=FALSE, "Unit"="", "Encoding"=enum."Discrete", "Default Value"="0"}, {"Core Number"=0, "Channel Number"=27, "Channel Name"="LGCS_MON2_TX", "Channel Speed"=100, "Label Decimal"=32, "Label Name"="Label_40", "Min Rate (mS)"=320, "Max Rate (mS)"=480, "SDI"=1, "SSM"=0, "Create SDI"=FALSE, "Create SSM"=FALSE, "Create Parity"=FALSE, "Parameter Name"="mlg1_lh_door_closed_prox_sensor_trend_mon_info_lsb51", "Start Bit"=21, "Number of Bits"=1, "Scale"="0", "Offset"="0", "Signed"=FALSE, "Unit"="", "Encoding"=enum."Discrete", "Default Value"="0"}, {"Core Number"=0, "Channel Number"=27, "Channel Name"="LGCS_MON2_TX", "Channel Speed"=100, "Label Decimal"=32, "Label Name"="Label_40", "Min Rate (mS)"=320, "Max Rate (mS)"=480, "SDI"=1, "SSM"=0, "Create SDI"=FALSE, "Create SSM"=FALSE, "Create Parity"=FALSE, "Parameter Name"="mlg1_lh_door_closed_prox_sensor_trend_mon_info_msb1", "Start Bit"=22, "Number of Bits"=1, "Scale"="0", "Offset"="0", 
